vi "Convert_Cycle_Info.vi"(0 "Converted Data In":T1 {"CRC" format="%04x"; "Length" format="%02x"; "Command" format="%02x"; "Destination" format="%02x"; "Source" format="%02x"}, 11 "Error In":errorcluster) -> (4 "Cycle Information":T2, 15 "Error Out":errorcluster)   [LabVIEW 2016]
uses:
  type defs/Cycle_Information.ctl
  Common/LabVIEW GEA2 Toolkit/LabVIEW_GEA2_Toolkit.lvlibp/type defs/Data Out.ctl
  Common/LabVIEW GEA2 Toolkit/LabVIEW_GEA2_Toolkit.lvlibp
panel:
  # "UI"
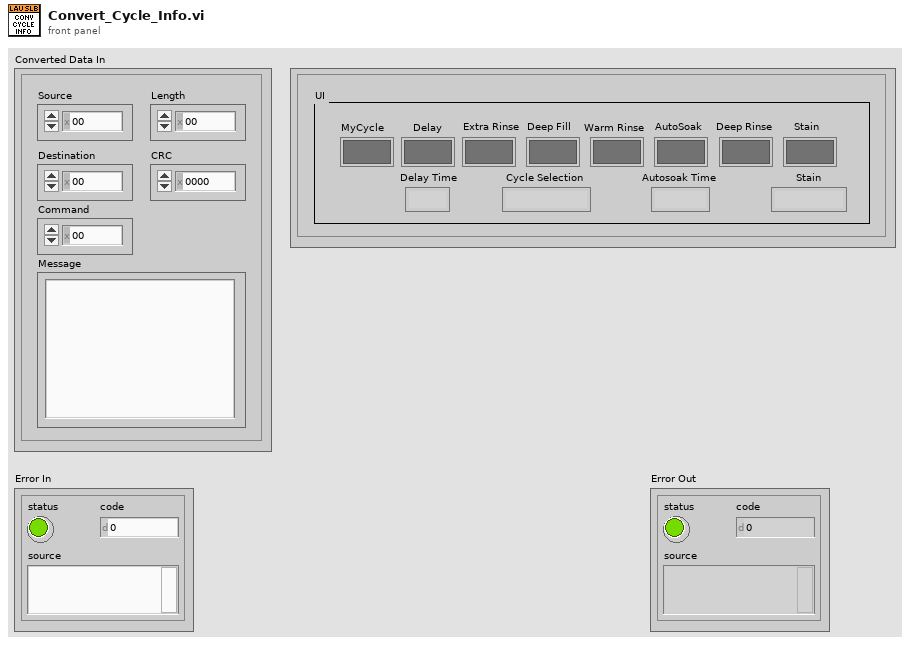
[diagram p1: front panel]
types:
  T1 = typedef "LabVIEW_GEA2_Toolkit.lvlibp/Data Out.ctl" = cluster{"Source":u8, "Destination":u8, "Command":u8, "Length":u8, "CRC":u16, "Message":string}
  T2 = typedef "Cycle_Information.ctl" = cluster{"MyCycle":bool, "Delay":bool, "Extra Rinse":bool, "Deep Fill":bool, "AutoSoak":bool, "Deep Rinse":bool, "Warm Rinse":bool, "Delay Time":string, "Stain":string, "Autosoak Time":string, "Cycle Selection":string, "Stain":bool}
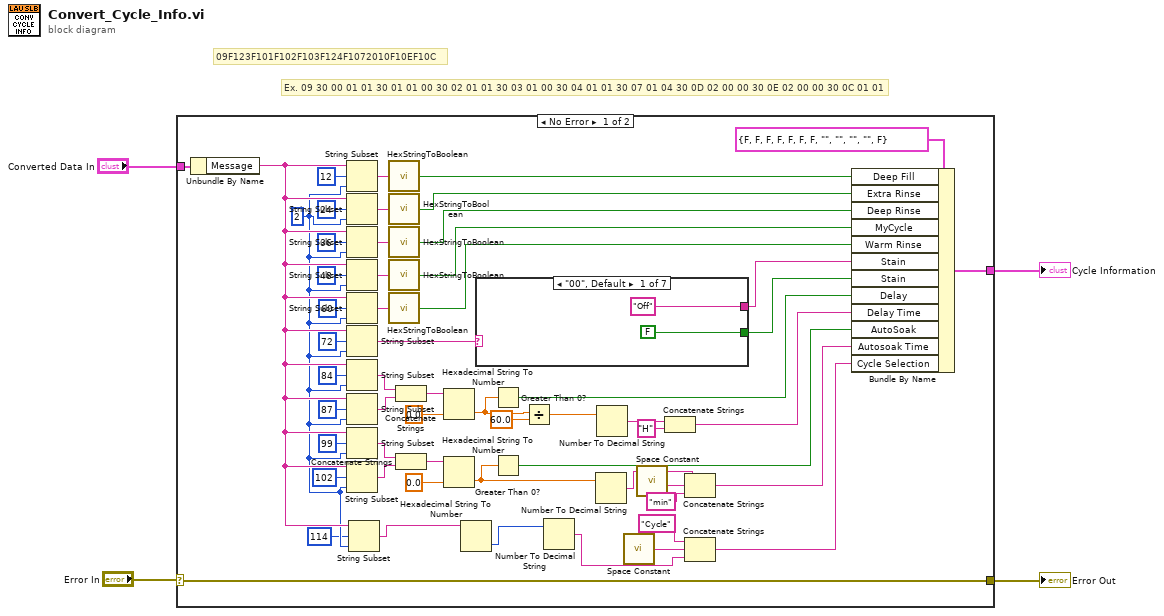
[diagram p0: block diagram]
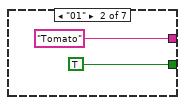
[diagram p2: hidden frame]
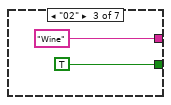
[diagram p3: hidden frame]
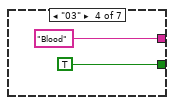
[diagram p4: hidden frame]
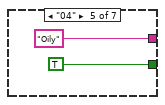
[diagram p5: hidden frame]
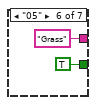
[diagram p6: hidden frame]
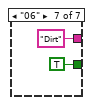
[diagram p7: hidden frame]
diagram:
  # "09F123F101F102F103F124F1072010F10EF10C"
  # "Ex. 09 30 00 01 01 30 01 01 00 30 02 01 01 30 03 01 00 30 04 01 01 30 07 01 04 30 0D 02 00 00 30 0E 02 00 00 30 0C 01 01"
  n1 = case shown="No Error" "Error In" {
    selector: "Error In" -> [w61 w76]
    tunnel: [w61 w76] -> w3
    tunnel: "Converted Data In" -> [w60 _]
    tunnel: [w32 _] -> w1
    frame No Error {
      w23 = 2 ("length (rest)")
      n2 = Unbundle By Name(w60) -> ("Message"=w24:string)
      n3 = String Subset(string=w24, offset (0)=12, length (rest)=w23) -> (substring=w52:string)
      n4 = String Subset(string=w24, offset (0)=24, length (rest)=w23) -> (substring=w49:string)
      n5 = String Subset(string=w24, offset (0)=36, length (rest)=w23) -> (substring=w46:string)
      n6 = String Subset(string=w24, offset (0)=48, length (rest)=w23) -> (substring=w48:string)
      n7 = String Subset(string=w24, offset (0)=60, length (rest)=w23) -> (substring=w47:string)
      n8 = String Subset(string=w24, offset (0)=72, length (rest)=w23) -> (substring=w41:string)
      n9 = String Subset(string=w24, offset (0)=84, length (rest)=w23) -> (substring=w37:string)
      n10 = String Subset(string=w24, offset (0)=87, length (rest)=w23) -> (substring=w36:string)
      n11 = String Subset(string=w24, offset (0)=99, length (rest)=w23) -> (substring=w29:string)
      n12 = String Subset(string=w24, offset (0)=102, length (rest)=w23) -> (substring=w25:string)
      n13 = String Subset(string=w24, offset (0)=114, length (rest)=w23) -> (substring=w21:string)
      n14 = call "HexStringToBoolean.vi"("Hex String"=w52) -> ("Boolean"=w50:bool)
      n15 = call "HexStringToBoolean.vi"("Hex String"=w49) -> ("Boolean"=w45:bool)
      n16 = call "HexStringToBoolean.vi"("Hex String"=w46) -> ("Boolean"=w44:bool)
      n17 = call "HexStringToBoolean.vi"("Hex String"=w48) -> ("Boolean"=w43:bool)
      n18 = call "HexStringToBoolean.vi"("Hex String"=w47) -> ("Boolean"=w42:bool)
      n19 = Concatenate Strings(w37, w36) -> (w34:string)
      n20 = Concatenate Strings(w29, w25) -> (w31:string)
      n21 = Hexadecimal String To Number(string=w34, default (0uL)=0.0) -> (number=w15:dbl)  [unwired: 1 in, 1 out]
      n22 = Hexadecimal String To Number(string=w31, default (0uL)=0.0) -> (number=w9:dbl)  [unwired: 1 in, 1 out]
      n23 = Hexadecimal String To Number(string=w21) -> (number=w20:u32)  [unwired: 2 in, 1 out]
      n24 = case shown="\"00\", Default" w41 {
        tunnel: [FALSE ("Stain Pretreat") TRUE ("Stain Pretreat") TRUE ("Stain Pretreat") TRUE ("Stain Pretreat") TRUE ("Stain Pretreat") TRUE ("Stain Pretreat") TRUE ("Stain Pretreat")] -> w39
        tunnel: ["Off" ("Stain") "Tomato" ("Stain") "Wine" ("Stain") "Blood" ("Stain") "Oily" ("Stain") "Grass" ("Stain") "Dirt" ("Stain")] -> w40
        frame "00", Default {
        }
        frame "01" {
        }
        frame "02" {
        }
        frame "03" {
        }
        frame "04" {
        }
        frame "05" {
        }
        frame "06" {
        }
      }
      n25 = Greater Than 0?(x=w15) -> (x > 0?=w33:bool)
      n26 = Greater Than 0?(x=w9) -> (x > 0?=w26:bool)
      n27 = Divide(x=w15, y=60.0) -> (x/y=w16:dbl)
      n28 = Number To Decimal String(number=w20) -> (decimal integer string=w13:string)  [unwired: 1 in]
      n29 = Number To Decimal String(number=w9) -> (decimal integer string=w8:string)  [unwired: 1 in]
      n30 = Number To Decimal String(number=w16) -> (decimal integer string=w19:string)  [unwired: 1 in]
      n31 = call <vilib>:"Space Constant.vi"() -> ("String"=w10:string)
      n32 = call <vilib>:"Space Constant.vi"() -> ("String"=w6:string)
      n33 = Concatenate Strings(w19, "H" ("string")) -> (w17:string)
      n34 = Concatenate Strings(w8, w6, "min" ("string")) -> (w5:string)
      n35 = Concatenate Strings("Cycle" ("string"), w10, w13) -> (w11:string)
      n36 = Bundle By Name(cluster=T2 {"MyCycle"=FALSE, "Delay"=FALSE, "Extra Rinse"=FALSE, "Deep Fill"=FALSE, "AutoSoak"=FALSE, "Deep Rinse"=FALSE, "Warm Rinse"=FALSE, "Delay Time"="", "Stain"="", "Autosoak Time"="", "Cycle Selection"="", "Stain"=FALSE} ("Cycle Information"), "Deep Fill"=w50, "Extra Rinse"=w45, "Deep Rinse"=w44, "MyCycle"=w43, "Warm Rinse"=w42, "Stain"=w40, "Stain"=w39, "Delay"=w33, "Delay Time"=w17, "AutoSoak"=w26, "Autosoak Time"=w5, "Cycle Selection"=w11) -> (w32:T2)
    }
    frame Error {
    }
  }
  "Error Out" <- w3
  "Cycle Information" <- w1
